vi "STP Request Response.vi"(8 "error in":errorcluster, 10 "Socket No":u16=1, 11 "STP Data in":T3={"ECU CAN Port"="CAN1", "CMD"=130, "CAN Write Data"=[], "Response Decoder"=enum."String", "String"={"Start Index"=0, "Length"=-1}, "Number"={"MSB Index"=0, "LSB Index"=1}, "Boolean"={"Index"=0, "Bool"={"7"=FALSE, "6"=FALSE, "5"=FALSE, "4"=FALSE, "3"=FALSE, "2"=FALSE, "1"=FALSE, "0"=FALSE, "7 Enabled"=FALSE, "6 Enabled"=FALSE, "5 Enabled"=FALSE, "4 Enabled"=FALSE, "3 Enabled"=FALSE, "2 Enabled"=FALSE, "1 Enabled"=FALSE, "0 Enabled"=FALSE}}} {"CMD" items=["TSW_VERSION(130)"=130, "WAIT_EVENT(132)"=132, "SEQUENCER(133)"=133, "TSW_RESET(150)"=150, "CONFIG_ECU(151)"=151, "TEST_CORE (152)"=152, "TEST_WATCHDOG (153)"=153, "TEST_MONITORING (154)"=154, "READ_MEMORY (162)"=162, "WRITE_ERASE_MEMORY (164)"=164, "COMM_EXTERNAL (190)"=190, "COMM_INTERNAL (195)"=195, "GET_ANALOG_INPUT (210)"=210, "GET_DIGITAL_INPUT (211)"=211, "GET_FREQUENCY_INPUT (212)"=212, "TEST_INPUT_STRUCTURE (214)"=214, "GENERATE_OUTPUT_SIGNAL (220)"=220, "GENERATE_SYNCHRONIZED_OUTPUT_SIGNALS (221)"=221, "eDCU_Specific (250)"=250]; "CAN Write Data" format="%.0x"}) -> (0 "error out":errorcluster, 1 "Report Text":string, 2 "STP Error":T2, 3 "STP Data Out":T1)   [LabVIEW 2023, in "HardwareAbstractionLayer_LVOOP.lvlib" / "Wait Monitor.lvclass"]
uses:
  Wait Monitor.lvclass
  Teststand Steptypes/CAN/STP/Steptypes/Control/STP Data.ctl
  CAN/CAN Application Protocols/STP Protocol_class/Ctrls/STP CMD.ctl
  CAN/CAN Application Protocols/STP Protocol_class/Ctrls/STP Error Cluster.ctl
  Teststand Steptypes/CAN/STP/Steptypes/Control/STP Out Data.ctl
  CAN/CAN Application Protocols/STP Protocol_class/Ctrls/STP Input Data.ctl
  CAN/CAN Application Protocols/STP Protocol_class/STP Protocol.lvclass
  Teststand Steptypes/LTT_TeststandSteptypes.lvlib
panel:
  # "Help : the index will choose the one element in an array and compare its true or false"
  # "Bit"
  # "Value"
  # "Enabled"
  # "Help : if the LSB index is -1 then it will take only MSB value"
  # "Help : if length -1 then it will take the entire array"
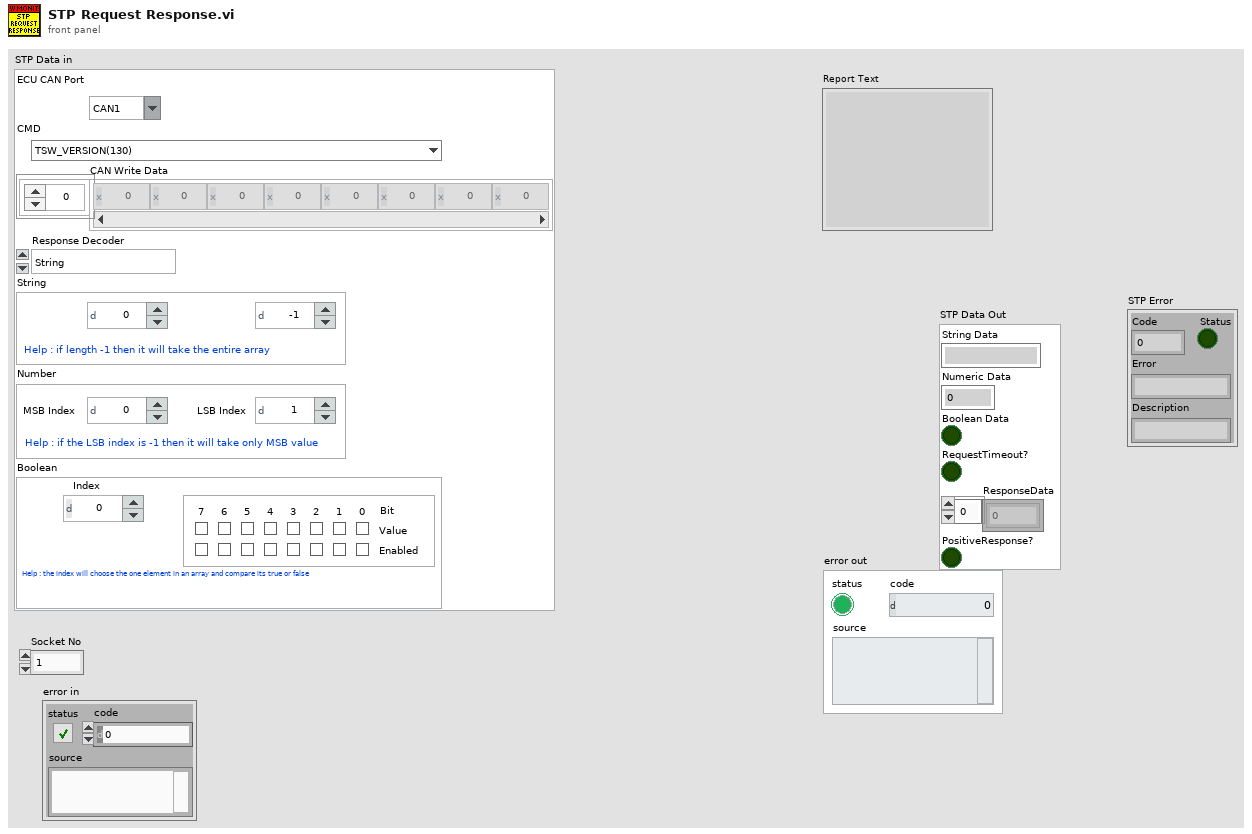
[diagram p1: front panel]
types:
  T1 = typedef "LTT_TeststandSteptypes.lvlib/STP Out Data.ctl" = cluster{"String Data":string, "Numeric Data":dbl, "Boolean Data":bool, "RequestTimeout?":bool, "ResponseData":u8[], "PositiveResponse?":bool}
  T2 = typedef "HardwareAbstractionLayer_LVOOP.lvlib/CAN Application Protocols Lib.lvlib/STP Protocol.lvclass/STP Error Cluster.ctl" = cluster{"Status":bool, "Code":u8, "Error":string, "Description":string}
  T3 = typedef "LTT_TeststandSteptypes.lvlib/STP Data.ctl" = cluster{"ECU CAN Port":string, "CMD":T4, "CAN Write Data":u8[], "Response Decoder":enum16{"String", "Number", "Boolean"}, "String":cluster{"Start Index":i32, "Length":i32}, "Number":cluster{"MSB Index":i32, "LSB Index":i32}, "Boolean":cluster{"Index":i32, "Bool":cluster{"7":bool, "6":bool, "5":bool, "4":bool, "3":bool, "2":bool, "1":bool, "0":bool, "7 Enabled":bool, "6 Enabled":bool, "5 Enabled":bool, "4 Enabled":bool, "3 Enabled":bool, "2 Enabled":bool, "1 Enabled":bool, "0 Enabled":bool}}}
  T4 = typedef "HardwareAbstractionLayer_LVOOP.lvlib/CAN Application Protocols Lib.lvlib/STP Protocol.lvclass/STP CMD.ctl" = u8
  T5 = typedef "HardwareAbstractionLayer_LVOOP.lvlib/CAN Application Protocols Lib.lvlib/STP Protocol.lvclass/STP Input Data.ctl" = cluster{"TxID":u32, "RxID":u32, "CMD":T4, "RQ Data":u8[], "+veResponseCode":u8, "ResponseTimeout (S)":dbl}
  T6 = typedef "HardwareAbstractionLayer_LVOOP.lvlib/CAN HAL Lib.lvlib/CAN.lvclass/CAN Init Ctrl.ctl" = cluster{"XNET Interface":refnum<k21>, "Baud Rate":u64, "CAN:Termination":u32, "Echo Transmit?":bool, "scope (normal)":T7}
  T7 = typedef "XNET Control Scope.ctl" = u32
  T8 = cluster{"Refnum out":refnum<k21>, "CAN Init Data":T6, "CAN_RxID":u32, "CAN_TxID":u32, "Timeout":dbl}
  T9 = typedef "HardwareAbstractionLayer_LVOOP.lvlib/CAN Application Protocols Lib.lvlib/STP Protocol.lvclass/STP Output Data.ctl" = cluster{"ResponseData":u8[], "ResponseData(ASCII)":string, "PositiveResponse?":bool, "STP Error":T2}
  T10 = cluster{"7":bool, "6":bool, "5":bool, "4":bool, "3":bool, "2":bool, "1":bool, "0":bool, "7 Enabled":bool, "6 Enabled":bool, "5 Enabled":bool, "4 Enabled":bool, "3 Enabled":bool, "2 Enabled":bool, "1 Enabled":bool, "0 Enabled":bool}
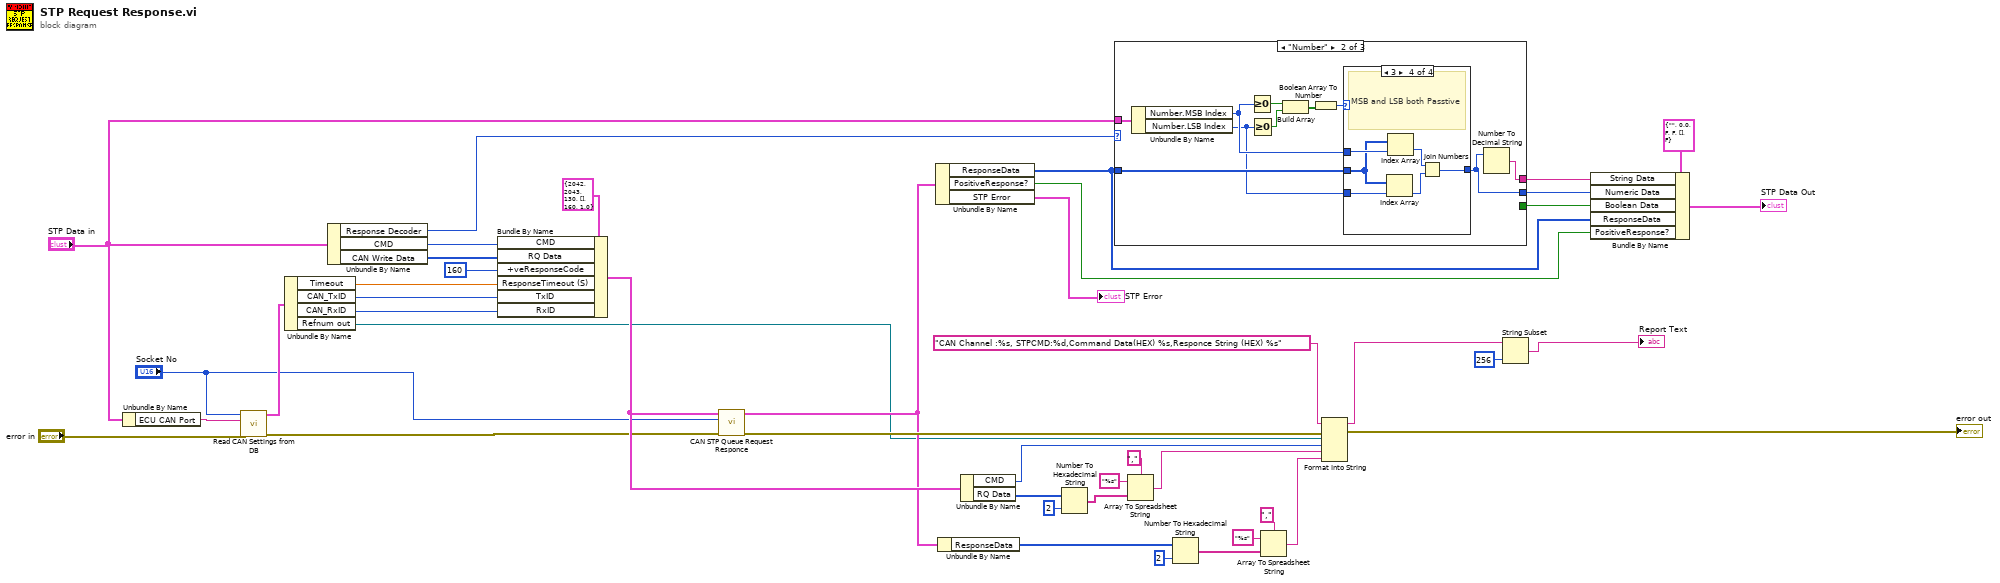
[diagram p0: block diagram]
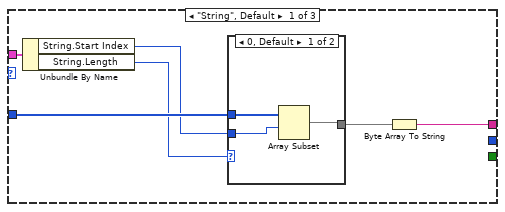
[diagram p2: hidden frame]
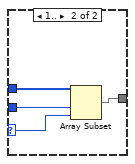
[diagram p3: hidden frame]
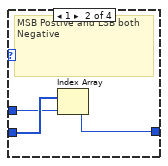
[diagram p5: hidden frame]
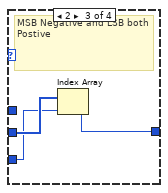
[diagram p6: hidden frame]
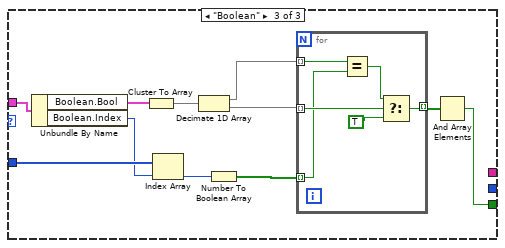
[diagram p7: hidden frame]
diagram:
  n1 = Unbundle By Name("STP Data in") -> ("ECU CAN Port"=w7:string)
  n2 = call "Read CAN Settings from DB.vi"("error in"="error in", "ECU CAN Port"=w7, "Socket No"="Socket No") -> ("error out"=w8:errorcluster, "Read CAN Setting"=w6:T8)  [unwired: 7 in]
  n3 = Unbundle By Name(w6) -> ("Timeout"=w5:dbl, "CAN_TxID"=w4:u32, "CAN_RxID"=w3:u32, "Refnum out"=w2:refnum<k21>)
  n4 = Unbundle By Name("STP Data in") -> ("Response Decoder"=w28:enum16{"String", "Number", "Boolean"}, "CMD"=w43:T4, "CAN Write Data"=w42:u8[])
  n5 = Bundle By Name(cluster=T5 {"TxID"=2042, "RxID"=2043, "CMD"=130, "RQ Data"=[], "+veResponseCode"=160, "ResponseTimeout (S)"=1.0} ("STP Input Data"), "CMD"=w43, "RQ Data"=w42, "+veResponseCode"=u8 160, "ResponseTimeout (S)"=w5, "TxID"=w4, "RxID"=w3) -> (w27:T5)
  n6 = call "CAN STP Queue Request Responce.vi"("error in (no error)"=w8, "Socket No"="Socket No", "STP Input Data"=w27) -> ("error out"=w29:errorcluster, "STP Output Data"=w22:T9)  [unwired: 6 in, 1 out]
  n7 = Unbundle By Name(w22) -> ("ResponseData"=w34:u8[], "PositiveResponse?"=w32:bool, "STP Error"=→"STP Error":T2)
  n8 = Unbundle By Name(w22) -> ("ResponseData"=w14:u8[])
  n9 = Unbundle By Name(w27) -> ("CMD"=w26:T4, "RQ Data"=w16:u8[])
  n10 = Number To Hexadecimal String(1:i16 2 ("width (-)"), 2:w16) -> (0:w20:string[])
  n11 = case shown="\"Number\"" w28 {
    tunnel: w34 -> [w49 w62 w87]
    tunnel: "STP Data in" -> [w50 w67 w90]
    tunnel: [w45 w58 _] -> w37
    tunnel: [_ w59 _] -> w36
    tunnel: [_ _ w80] -> w35
    frame "String", Default {
      n12 = Unbundle By Name(w50) -> ("String.Start Index"=w48:i32, "String.Length"=w47:i32)
      n13 = case shown="0, Default" w47 {
        selector: w47 -> [_ w55]
        tunnel: w49 -> [w53 w57]
        tunnel: w48 -> [w52 w56]
        tunnel: [w51 w54] -> w46
        frame 0, Default {
          n14 = Array Subset(array=w53, index=w52) -> (w51:u8[])  [unwired: 1 in]
        }
        frame 1.. {
          n15 = Array Subset(array=w57, index=w56, length=w55) -> (w54:u8[])
        }
      }
      n16 = Byte Array To String(unsigned byte array=w46) -> (string=w45:string)
    }
    frame "Number" {
      n17 = Unbundle By Name(w67) -> ("Number.MSB Index"=w61:i32, "Number.LSB Index"=w60:i32)
      n18 = Greater Or Equal To 0?(x=w61) -> (x >= 0?=w66:bool)
      n19 = Greater Or Equal To 0?(x=w60) -> (x >= 0?=w65:bool)
      n20 = Build Array(w66, w65) -> (w64:bool[])
      n21 = Boolean Array To Number(Boolean array=w64) -> (number=w63:u32)
      n22 = case shown="3" w63 {
        tunnel: w62 -> [_ w70 w73 w78]
        tunnel: w61 -> [_ w69 _ w79]
        tunnel: w60 -> [_ _ w71 w77]
        tunnel: [_ w68 w72 w74] -> w59
        frame 0, Default {
          # "MSB and LSB both Negative"
        }
        frame 1 {
          # "MSB Postive and LSB both Negative"
          n23 = Index Array(array=w70, index=w69) -> (element=w68:u8)
        }
        frame 2 {
          # "MSB Negative and LSB both Postive"
          n24 = Index Array(array=w73, index=w71) -> (element=w72:u8)
        }
        frame 3 {
          # "MSB and LSB both Passtive"
          n25 = Index Array(array=w78, index=w77) -> (element=w75:u8)
          n26 = Index Array(array=w78, index=w79) -> (element=w76:u8)
          n27 = Join Numbers(hi=w76, lo=w75) -> ((hi.lo)=w74:u16)
        }
      }
      n28 = Number To Decimal String(number=w59) -> (decimal integer string=w58:string)  [unwired: 1 in]
    }
    frame "Boolean" {
      n29 = Unbundle By Name(w90) -> ("Boolean.Bool"=w89:T10, "Boolean.Index"=w86:i32)
      n30 = Cluster To Array(cluster=w89) -> (array=w88:bool[])
      n31 = Index Array(array=w87, index=w86) -> (element=w85:u8)
      n32 = Decimate 1D Array(w88) -> (w83:bool[], w82:bool[])
      n33 = Number To Boolean Array(number=w85) -> (Boolean array=w84:bool[])
      n34 = for {
        tunnel: w84 -> [w94] mode=indexing
        tunnel: w83 -> [w95] mode=indexing
        tunnel: w82 -> [w96] mode=indexing
        tunnel: [w91] -> w81 mode=indexing
        n35 = Equal?(x=w95, y=w94) -> (x = y?=w93:bool)
        n36 = Select(t=w93, s=w96, f=TRUE) -> (s? t:f=w91:bool)
      }
      n37 = And Array Elements(Boolean array=w81) -> (logical AND=w80:bool)
    }
  }
  n38 = Array To Spreadsheet String(delimiter (Tab)=",", array=w20, 3:"%s" ("format string")) -> (spreadsheet string=w24:string)
  n39 = Number To Hexadecimal String(1:i16 2 ("width (-)"), 2:w14) -> (0:w13:string[])
  n40 = Array To Spreadsheet String(delimiter (Tab)=",", array=w13, 3:"%s" ("format string")) -> (spreadsheet string=w12:string)
  n41 = Format Into String(format string="CAN Channel :%s, STPCMD:%d,Command Data(HEX) %s,Responce String (HEX) %s", error in=w29, w2, w26, w24, w12) -> (resulting string=w11:string, error out=→"error out":errorcluster)  [unwired: 1 in]
  n42 = String Subset(string=w11, length (rest)=256 ("length (rest)")) -> (substring=→"Report Text":string)  [unwired: 1 in]
  n43 = Bundle By Name(cluster=T1 {"String Data"="", "Numeric Data"=0.0, "Boolean Data"=FALSE, "RequestTimeout?"=FALSE, "ResponseData"=[], "PositiveResponse?"=FALSE} ("STP Data Out"), "String Data"=w37, "Numeric Data"=w36, "Boolean Data"=w35, "ResponseData"=w34, "PositiveResponse?"=w32) -> (→"STP Data Out":T1)
